vi "OSF Create Component.vi"(7 "OSF API URL":string="https://api.osf.io/v2/", 8 "error in":errorcluster, 9 "Child name":string, 10 "Parent  ID":string, 11 "client handle":T2) -> (0 "error out":errorcluster, 2 "Component ID":string caption="Project ID", 3 "client handle out":T2)   [LabVIEW 2020]
uses:
  <vilib>/httpClient/ClientHandle.ctl
  55103850-15ef-4a18-9388-7b0eadcdd449.vi
  <vilib>/JDP Science/JSONtext/Variant to JSON Text.vi
  <vilib>/httpClient/POSTBuffer.vi
  <vilib>/JDP Science/JSONtext/LVClass Serializer/JSONtext LVClass Serializer.lvclass
  <vilib>/httpClient/LabVIEWHTTPClient.lvlib
  <vilib>/JDP Science/JSONtext/JSONtext.lvlib
panel:
  out "Responce":string
  in  "OSF child":T1={"data"={"type"="nodes", "attributes"={"title"="", "description"="", "public"=FALSE, "category"="project"}}}
  out "Project  JSON":string
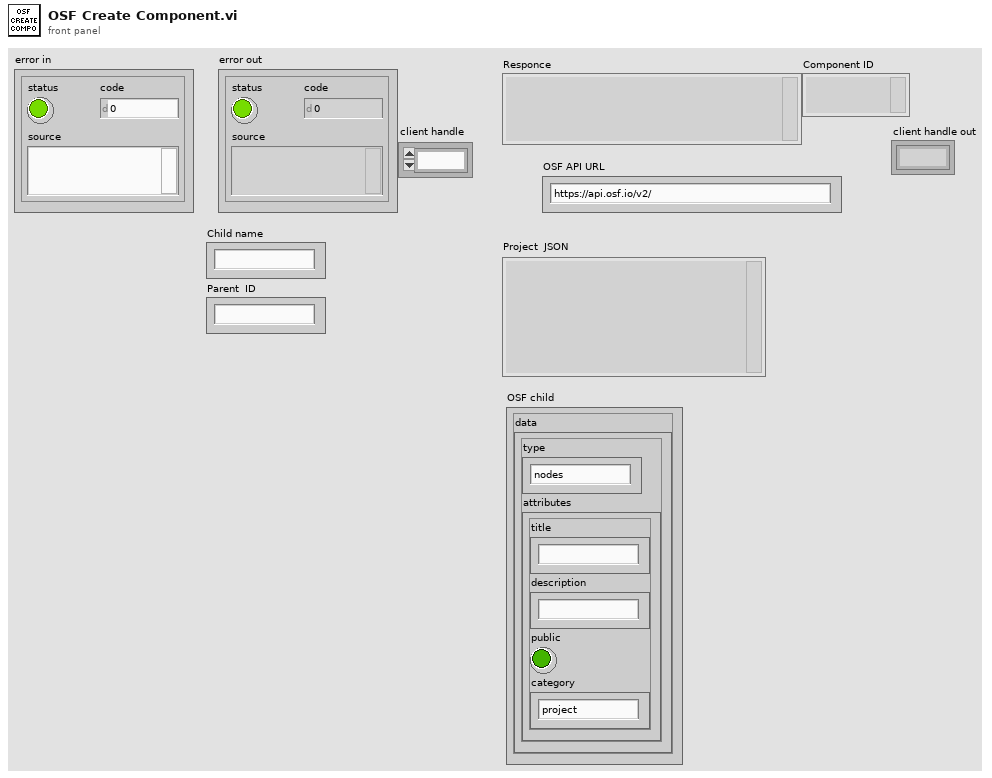
[diagram p1: front panel]
types:
  T1 = cluster{"data":cluster{"type":string, "attributes":cluster{"title":string, "description":string, "public":bool, "category":string}}}
  T2 = typedef "LabVIEWHTTPClient.lvlib/ClientHandle.ctl" = refnum<k1>
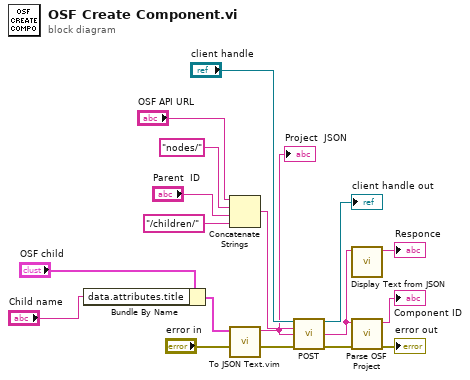
[diagram p0: block diagram]
diagram:
  n1 = Bundle By Name(cluster="OSF child", "data.attributes.title"="Child name") -> (w18:T1)
  n2 = Concatenate Strings("OSF API URL", "nodes/", "Parent  ID", "/children/" ("string")) -> (w9:string)
  n3 = call "To JSON Text.vim"("error in (no error)"="error in", "Anything"=w18) -> ("error out"=w8:errorcluster, "<JSON>"=w6:string)  [unwired: 8 in]
  "Project  JSON" <- w6
  n4 = call-poly <vilib>:"POST.vi"("client handle"="client handle", "url"=w9, "buffer"=w6, "error in (no error)"=w8) -> ("client handle out"=→"client handle out":T2, "body"=w2:string, "error out"=w5:errorcluster)  [unwired: 8 in, 1 out]
  n5 = call <vilib>:"Display Text from JSON.vi"("Input JSON"=w2) -> ("Display Text"=→"Responce":string)  [unwired: 8 in, 2 out]
  n6 = call "Parse OSF Project.vi"("error in"=w5, "Project JSON"=w2) -> ("error out"=→"error out":errorcluster, "Project ID"=→"Component ID":string)  [unwired: 7 in, 1 out]
